vi "Close.vi"(8 "error in (no error)":errorcluster, 11 "Ismatech Settings":T1={"VISA resource name"="", "Simulated?"=FALSE, "Pump Number"=1.0, "Reverse?"=FALSE} {"Pump Number" min=1.0 max=20.0 step=1.0}) -> (0 "error out":errorcluster, 1 "Connection Error":bool, 3 "Ismatech Settings":T1={"VISA resource name"="", "Simulated?"=FALSE, "Pump Number"=1.0, "Reverse?"=FALSE} {"Pump Number" min=1.0 max=20.0 step=1.0})   [LabVIEW 2021, in "Ismatec ISM 831C.lvlib"]
uses:
  Ismatec ISM 831C.lvlib
  Controls/Ismatech ISM831C Settings Cluster.ctl
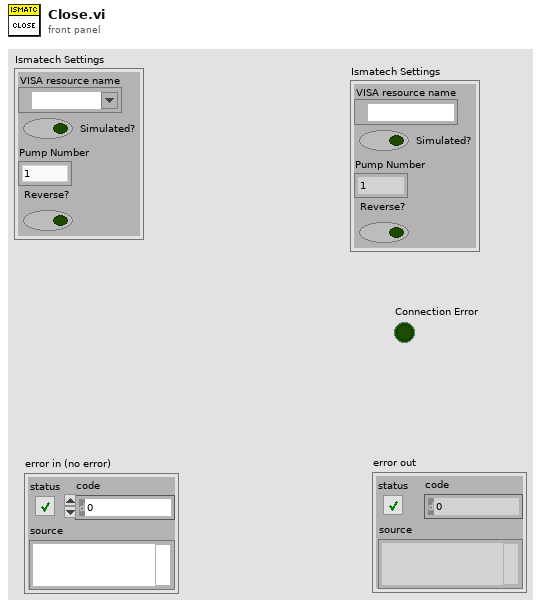
[diagram p1: front panel]
types:
  T1 = typedef "Ismatec ISM 831C.lvlib/Ismatech ISM831C Settings Cluster.ctl" = cluster{"VISA resource name":refnum<visa-resource-name>, "Simulated?":bool, "Pump Number":dbl, "Reverse?":bool}
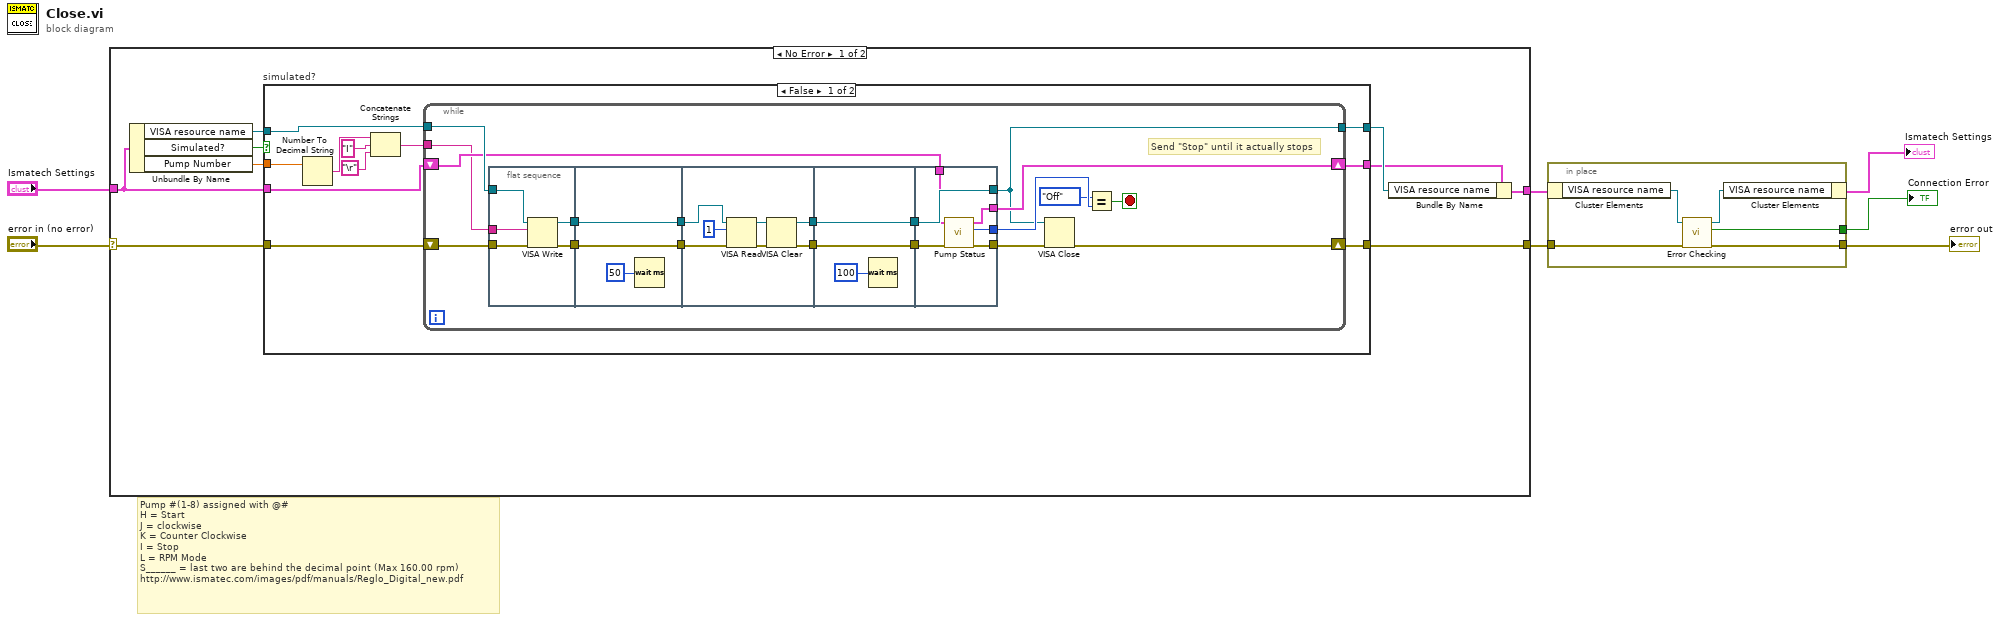
[diagram p0: block diagram]
diagram:
  # "Pump #(1-8) assigned with @#\nH = Start\nJ = clockwise\nK = Counter Clockwise\nI = Stop\nL = RPM Mode\nS______ = last two are behind the decimal point (Max 160.00 rpm)\nhttp://www.ismatec.com/images/pdf/manuals/Reglo_Digital_new.pdf"
  n1 = case shown="No Error" "error in (no error)" {
    selector: "error in (no error)" -> [w11 w75]
    tunnel: [w15 w75] -> w5
    tunnel: [w12 w74] -> w2
    tunnel: "Ismatech Settings" -> [w8 w74]
    frame No Error {
      n2 = Unbundle By Name(w8) -> ("VISA resource name"=w10:refnum<visa-resource-name>, "Simulated?"=w16:bool, "Pump Number"=w13:dbl)
      n3 = case "simulated?" shown="False" w16 {
        tunnel: [w27 w71] -> w15
        tunnel: [w22 w72] -> w14
        tunnel: w13 -> [w20 _]
        tunnel: w11 -> [w26 w71]
        tunnel: w10 -> [w25 w72]
        tunnel: w8 -> [w24 w73]
        tunnel: [w23 w73] -> w9
        frame False {
          n4 = Number To Decimal String(number=w20) -> (decimal integer string=w21:string)  [unwired: 1 in]
          n5 = Concatenate Strings(w21, "I" ("string"), "\r") -> (w17:string)
          n6 = while {
            tunnel: w25 -> [w35]
            shift-right: [w38] -> w27
            shift-left: w26 -> [w36]
            shift-right: [w33] -> w23
            shift-left: w24 -> [w34]
            tunnel: [w30] -> w22
            tunnel: w17 -> [w28]
            stop <- w32 stop-if-true
            # "Send \"Stop\" until it actually stops"
            n7 = flat-sequence {
              tunnel: w36 -> [w51]
              tunnel: w35 -> [w50]
              tunnel: [w49] -> w46
              tunnel: [w48] -> w45
              tunnel: w28 -> [w47]
              tunnel: [w53] -> w44
              tunnel: w46 -> [w53]
              tunnel: w45 -> [w52]
              tunnel: [w52] -> w43
              tunnel: w44 -> [w56]
              tunnel: w43 -> [w55]
              tunnel: [w58] -> w42
              tunnel: [w57] -> w41
              tunnel: w42 -> [w64]
              tunnel: w41 -> [w63]
              tunnel: [w64] -> w40
              tunnel: [w63] -> w39
              tunnel: [w68] -> w37
              tunnel: [w70] -> w30
              tunnel: w40 -> [w70]
              tunnel: w39 -> [w69]
              tunnel: w34 -> [w67]
              tunnel: [w66] -> w33
              tunnel: [w65] -> w31
              frame #0 {
                n8 = VISA Write(VISA resource name=w50, write buffer=w47, error in (no error)=w51) -> (VISA resource name out=w49:refnum<visa-resource-name>, error out=w48:errorcluster)  [unwired: 1 out]
              }
              frame #1 {
                n9 = Wait (ms)(milliseconds to wait=u32 50) -> ()  [unwired: 1 out]
              }
              frame #2 {
                n10 = VISA Read(VISA resource name=w56, byte count=u32 1, error in (no error)=w55) -> (VISA resource name out=w60:refnum<visa-resource-name>, error out=w61:errorcluster)  [unwired: 2 out]
                n11 = VISA Clear(VISA resource name=w60, error in (no error)=w61) -> (VISA resource name out=w58:refnum<visa-resource-name>, error out=w57:errorcluster)
              }
              frame #3 {
                n12 = Wait (ms)(milliseconds to wait=u32 100) -> ()  [unwired: 1 out]
              }
              frame #4 {
                n13 = call "Pump Status.vi"("error in (no error)"=w69, "Ismatech Settings In"=w67) -> ("error out"=w68:errorcluster, "Pump On?"=w65:enum16{"Off", "On", "Not Initialized"}, "Ismatech Settings Out"=w66:T1)  [unwired: 6 in, 1 out]
              }
            }
            n14 = VISA Close(VISA resource name=w30, error in (no error)=w37) -> (error out=w38:errorcluster)
            n15 = Equal?(x=enum16{"Off", "On", "Not Initialized"}."Off", y=w31) -> (x = y?=w32:bool)
          }
        }
        frame True {
        }
      }
      n16 = Bundle By Name(cluster=w9, "VISA resource name"=w14) -> (w12:T1)
    }
    frame Error {
    }
  }
  n17 = in-place {
    in-place-border: w5 -> [w80]
    in-place-border: [w79] -> w4
    in-place-border: [w78] -> w3
    n18 = in-place-cluster #1(w2) -> ("VISA resource name"=w77:refnum<visa-resource-name>)
    n19 = call "Error Checking.vi"("error in (no error)"=w80, "VISA resource name"=w77) -> ("error out"=w79:errorcluster, "Connection Error"=w78:bool, "VISA resource name"=w76:refnum<visa-resource-name>)  [unwired: 7 in]
    n20 = in-place-cluster #1("VISA resource name"=w76) -> (→"Ismatech Settings":T1)
  }
  "error out" <- w4
  "Connection Error" <- w3
